vi "Recurse.vi"(8 "Error in":errorcluster, 10 "Msg DVR in":refnum<data-value>, 11 "Base Actor in":refnum<class "Base Actor.lvclass">) -> (0 "Error out":errorcluster, 2 "Msg DVR out":refnum<data-value>, 3 "Base Actor out":refnum<class "Base Actor.lvclass">)   [LabVIEW 2020, in "jettl.lvlib" / "BaseActor.lvlib" / "Base Actor.lvclass"]
uses:
  Base Actor.lvclass
  Base Actor.lvclass/Base Actor.ctl
  ActorRelation.ctl
  jettl.lvlib
  MessageMetadata.ctl
  Message.ctl
  Message/Message.lvclass
  ActorLifetime.ctl
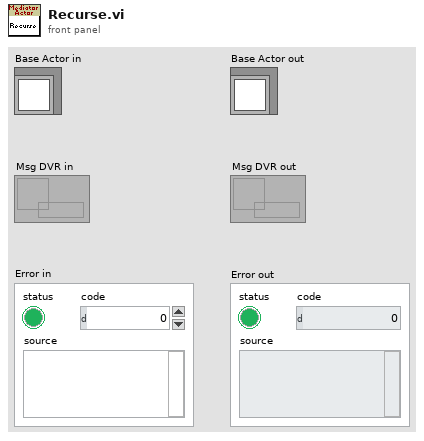
[diagram p1: front panel]
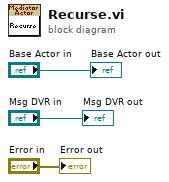
[diagram p0: block diagram]
diagram:
  "Base Actor out" <- "Base Actor in"
  "Error out" <- "Error in"
  "Msg DVR out" <- "Msg DVR in"
